vi "svi_write_ext_in.vi"(4 "shutter en entrée":bool, 5 "position num":u32, 6 "power value":dbl, 7 "pdir_path":path, 8 "shutter 1":bool, 9 "z value":dbl, 10 "power value 2":dbl, 11 "chanel num":u8) -> (0 "sortie d'erreur":errorcluster)   [LabVIEW 2013]
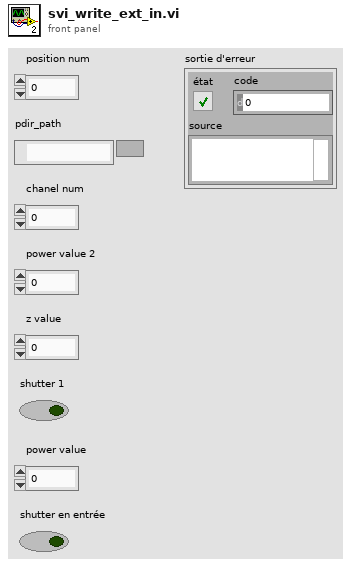
[diagram p1: front panel]
types:
  T1 = enum16{"open", "replace", "create", "open or create", "replace or create", "replace or create with confirmation"}
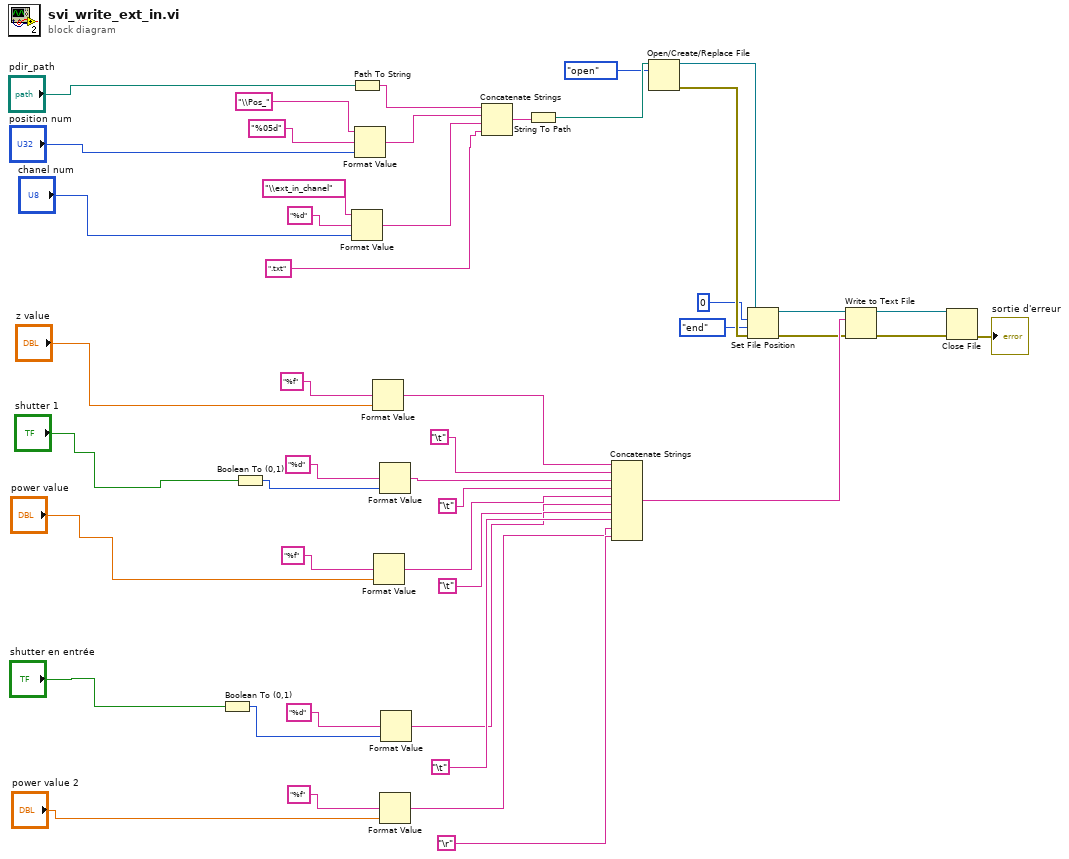
[diagram p0: block diagram]
diagram:
  n1 = Boolean To (0,1)(Boolean="shutter en entrée") -> (0, 1=w37:i16)
  n2 = Boolean To (0,1)(Boolean="shutter 1") -> (0, 1=w38:i16)
  n3 = Path To String(path="pdir_path") -> (string=w12:string)
  n4 = Format Value(string ("")="\\ext_in_chanel", format string="%d" ("chaîne"), value (0)="chanel num") -> (output string=w14:string)
  n5 = Format Value(string ("")="\\Pos_", format string="%05d" ("chaîne"), value (0)="position num") -> (output string=w13:string)
  n6 = Format Value(format string="%f" ("chaîne"), value (0)="z value") -> (output string=w32:string)  [unwired: 1 in]
  n7 = Format Value(format string="%f" ("chaîne"), value (0)="power value") -> (output string=w40:string)  [unwired: 1 in]
  n8 = Format Value(format string="%d" ("chaîne"), value (0)=w38) -> (output string=w34:string)  [unwired: 1 in]
  n9 = Format Value(format string="%f" ("chaîne"), value (0)="power value 2") -> (output string=w44:string)  [unwired: 1 in]
  n10 = Format Value(format string="%d" ("chaîne"), value (0)=w37) -> (output string=w42:string)  [unwired: 1 in]
  n11 = Concatenate Strings(w12, w13, w14, ".txt") -> (w17:string)
  n12 = String To Path(string=w17) -> (path=w18:path)
  n13 = Concatenate Strings(w32, "\t", w34, "\t", w40, "\t", w42, "\t", w44, "\r") -> (w36:string)
  n14 = Open/Create/Replace File(file path (use dialog)=w18, operation (0:open)=T1."open") -> (refnum out=w21:refnum<file>, error out=w22:errorcluster)  [unwired: 4 in, 1 out]
  n15 = Set File Position(offset (in bytes) (0)=i64 0, refnum=w21, from (0:start)=enum16{"start", "end", "current"}."end", error in=w22) -> (refnum out=w24:refnum<file>, error out=w23:errorcluster)
  n16 = Write to Text File(file (use dialog)=w24, text=w36, error in=w23) -> (refnum out=w25:refnum<file>, error out=w26:errorcluster)  [unwired: 1 in, 1 out]
  n17 = Close File(refnum=w25, error in=w26) -> (error out=→"sortie d'erreur":errorcluster)  [unwired: 1 out]
